vi "L_Layer_Model.vi"(2 "verbose":i32=1 min=1, 3 "num_iterations":i32, 4 "learning_rate":dbl, 5 "layer_dims":i32[](array[numeric]), 6 "Y":dbl[][](array[numeric]), 7 "X":dbl[][](array[numeric])) -> (0 "accuracy & loss":cluster{"Accuracy":dbl, "loss":dbl}[](array[cluster]), 1 "train_params":map{string, dbl[][]}(c390))   [LabVIEW 2020]
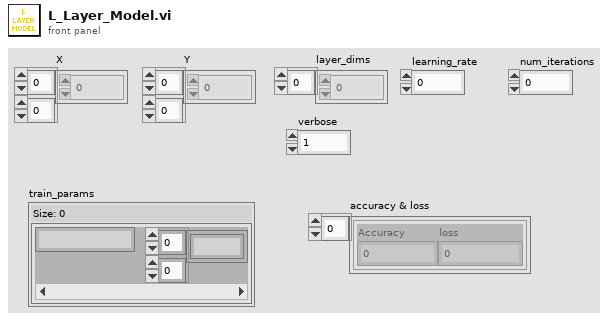
[diagram p1: front panel]
types:
  T1 = cluster{"A":dbl[][], "W":dbl[][], "b":dbl[][], "Z":dbl[][]}[]
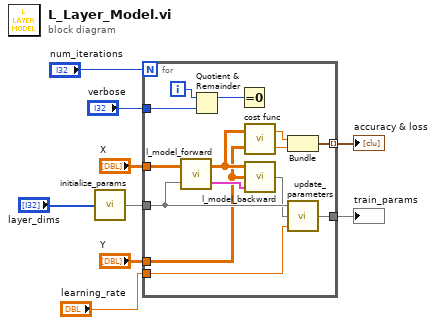
[diagram p0: block diagram]
diagram:
  n1 = call "initialize_params.vi"("layer_nodes"="layer_dims") -> ("parameters"=w7:map{string, dbl[][]})
  n2 = for {
    N: "num_iterations" -> [_]
    tunnel: w7 -> [w21]
    tunnel: "X" -> [w23]
    tunnel: "Y" -> [w16]
    tunnel: "learning_rate" -> [w19]
    tunnel: [w18] -> w3
    tunnel: "verbose" -> [w14]
    tunnel: [w10] -> w1 mode=indexing
    i -> [w15]
    n3 = call "l_model_forward.vi"("parameters"=w21, "X"=w23) -> ("caches"=w22:T1, "AL"=w17:dbl[][])
    n4 = Quotient & Remainder(x=w15, y=w14) -> (x-y*floor(x/y)=w13:i32)  [unwired: 1 out]
    n5 = Equal To 0?(x=w13) -> ()  [unwired: 1 out]
    n6 = call "cost func.vi"("Y"=w16, "AL"=w17) -> ("loss"=w11:dbl, "Accuracy"=w12:dbl)
    n7 = call "l_model_backward.vi"("caches"=w22, "Y"=w16, "AL"=w17) -> ("grads"=w20:map{string, dbl[][]})
    n8 = Bundle("Accuracy"=w12, "loss"=w11) -> (w10:cluster{"Accuracy":dbl, "loss":dbl})  [unwired: 1 in]
    n9 = call "update_parameters.vi"("learning_rate"=w19, "grads"=w20, "parameters"=w21) -> ("train_params"=w18:map{string, dbl[][]})
  }
  "train_params" <- w3
  "accuracy & loss" <- w1
